vi "Encoder Quad Phase Detection.vi"(6 "direzione":bool, 8 "Phase B":bool, 9 "Phase A":bool, 10 "Clear Error?":bool, 11 "Enable?":bool) -> (1 "Signal":bool, 2 "Backward?":bool, 3 "Error":bool, 4 "deltaT":i32)   [LabVIEW 2017]
uses:
  Encoder States.ctl
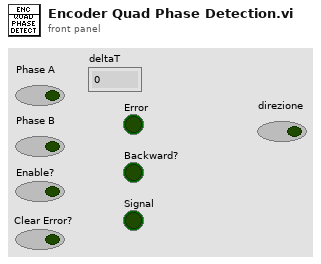
[diagram p1: front panel]
types:
  T1 = typedef "Encoder States.ctl" = fxp<+,3,3>
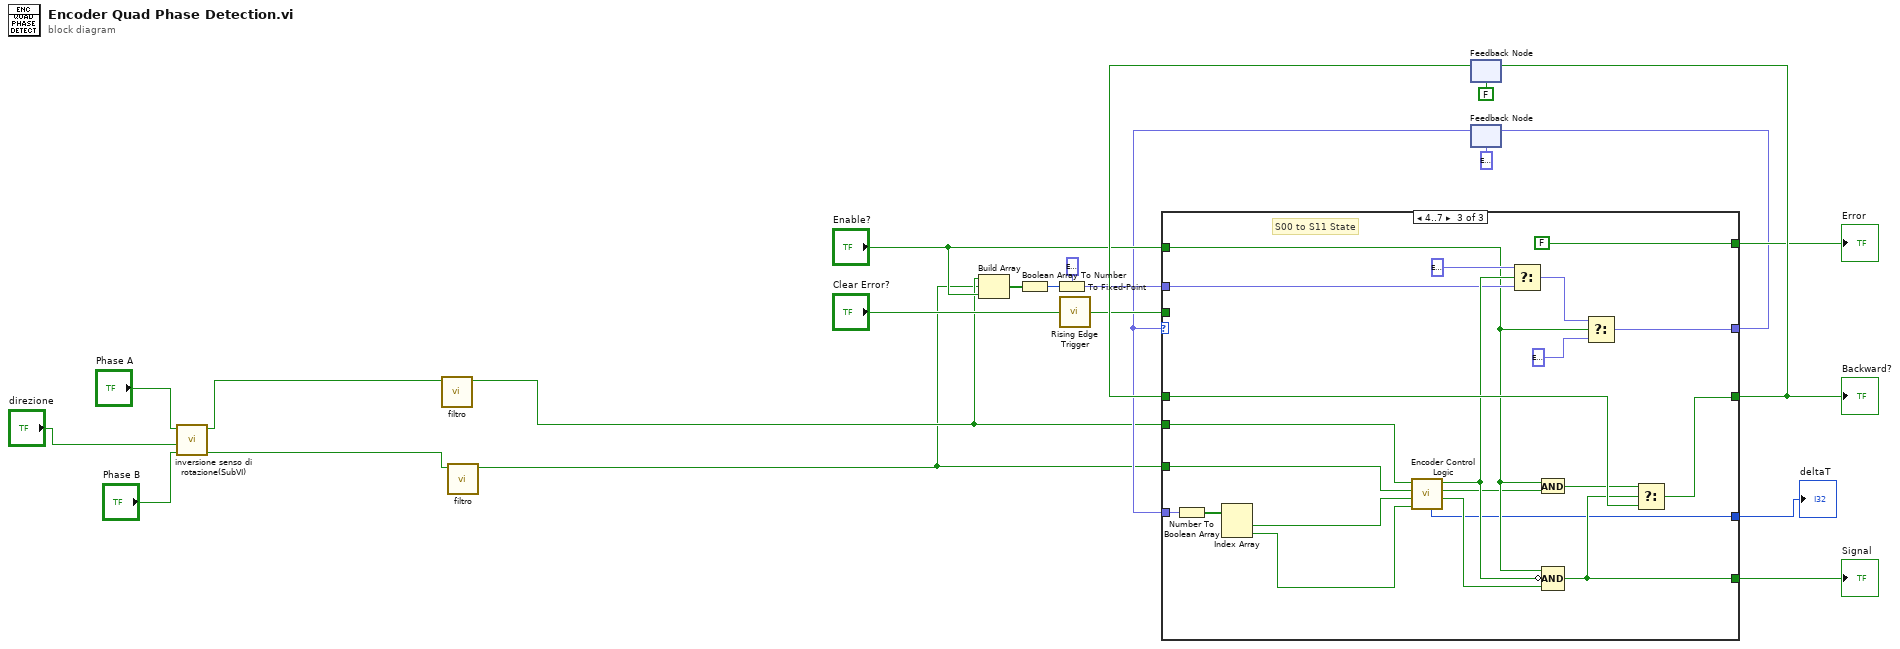
[diagram p0: block diagram]
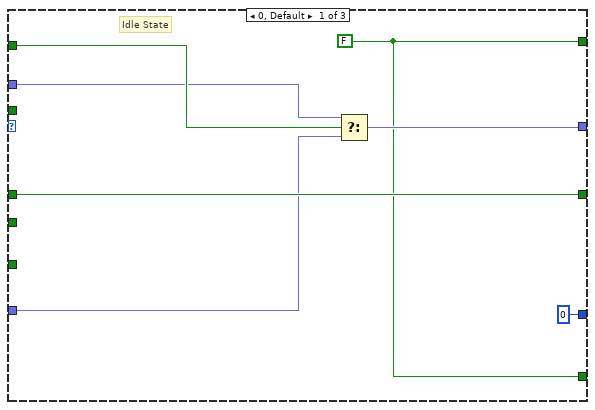
[diagram p2: hidden frame]
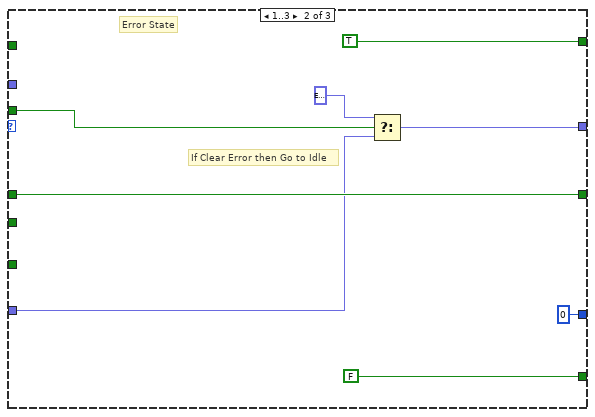
[diagram p3: hidden frame]
diagram:
  n1 = call "inversione senso di rotazione(SubVI).vi"("Boolean in 2"="Phase B", "VersoOrarioM1"="direzione", "Boolean in 1"="Phase A") -> ("Boolean out 2"=w2:bool, "Boolean out 1"=w4:bool)  [unwired: 5 in]
  n2 = call "filtro.vi"("Boolean out 1"=w4) -> ("Boolean"=w3:bool)  [unwired: 10 in]
  n3 = call "filtro.vi"("Boolean out 1"=w2) -> ("Boolean"=w1:bool)  [unwired: 10 in]
  n4 = Build Array(w3, w1, "Enable?") -> (w12:bool[])
  n5 = Boolean Array To Number(Boolean array=w12) -> (number=w11:u8)
  n6 = To Fixed-Point(fixed-point type=T1 0.0 ("Numeric"), number=w11) -> (fixed-point=w9:T1)
  n7 = call "Rising Edge Trigger.vi"("Signal"="Clear Error?") -> ("Trigger?"=w15:bool)
  n8 = feedback #1(FALSE ("Direction")) -> (w17:bool)
  n9 = feedback #2(T1 0.0) -> (w13:T1)
  n10 = case shown="4..7" w13 {
    tunnel: "Enable?" -> [w30 _ w46]
    tunnel: [w28 w35 w50] -> w19
    tunnel: [w26 TRUE ("Error") FALSE ("Error")] -> w21
    tunnel: w9 -> [w29 _ w54]
    tunnel: w17 -> [w27 w37 w59]
    tunnel: [w27 w37 w58] -> w22
    tunnel: [w26 FALSE ("Error") w48] -> w23
    tunnel: w15 -> [_ w36 _]
    tunnel: w1 -> [_ _ w56]
    tunnel: w3 -> [_ _ w57]
    tunnel: w13 -> [w25 w32 w41]
    tunnel: [0 ("deltaT") 0 ("deltaT") w39] -> w8
    frame 0, Default {
      w26 = FALSE ("Error")
      # "Idle State"
      n11 = Select(t=w29, s=w30, f=w25) -> (s? t:f=w28:T1)
    }
    frame 1..3 {
      # "Error State"
      # "If Clear Error then Go to Idle"
      n12 = Select(t=T1 0.0, s=w36, f=w32) -> (s? t:f=w35:T1)
    }
    frame 4..7 {
      # "S00 to S11 State"
      n13 = Number To Boolean Array(number=w41) -> (Boolean array=w43:bool[])
      n14 = Index Array(array=w43) -> (element #1=w42:bool, element #2=w40:bool)  [unwired: 2 in]
      n15 = call "Encoder Control Logic.vi"("Prev Phase B (State Bit 1)"=w40, "Prev Phase A (State Bit 0)"=w42, "Phase B"=w56, "Phase A"=w57) -> ("Count?"=w45:bool, "Backward?"=w44:bool, "Error Occurred?"=w55:bool, "deltaT"=w39:i32)  [unwired: 4 in]
      n16 = Select(t=T1 4.0, s=w55, f=w54) -> (s? t:f=w52:T1)
      n17 = And(x=w46, y=w44) -> (x .and. y?=w47:bool)
      n18 = Compound Arithmetic op=AND(w46, invert w55, w45) -> (w48:bool)
      n19 = Select(t=w52, s=w46, f=T1 0.0) -> (s? t:f=w50:T1)
      n20 = Select(t=w47, s=w48, f=w59) -> (s? t:f=w58:bool)
    }
  }
  "Backward?" <- w22
  "Signal" <- w23
  "Error" <- w21
  "deltaT" <- w8
  n21 = feedback-in #1(w22) -> ()
  n22 = feedback-in #2(w19) -> ()
